vi "ScalePitchCtrl.vi"(6 "Scale Direction":T3=enum."Full scale -> Model scale", 8 "Scale Factor":dbl, 11 "PitchCtrl (In)":T1={"P-Gain"=0.0, "Blade pitch operating mode"=enum."From File", "Constant setpoint (deg)"=0.0, "I-Gain"=0.0, "Pitch from File (deg)"=0.0, "Homing vel (rpm)"=0.0, "Max vel (rpm)"=0.0, "Max vel change (rpm/min)"=0.0}) -> (3 "PitchCtrl (Out)":T1={"P-Gain"=0.0, "Blade pitch operating mode"=enum."From File", "Constant setpoint (deg)"=0.0, "I-Gain"=0.0, "Pitch from File (deg)"=0.0, "Homing vel (rpm)"=0.0, "Max vel (rpm)"=0.0, "Max vel change (rpm/min)"=0.0})   [LabVIEW 2018]
uses:
  Clusters/ScalingEnum.ctl
  Clusters/PitchCtrl.ctl
  Clusters/BladePitchMode.ctl
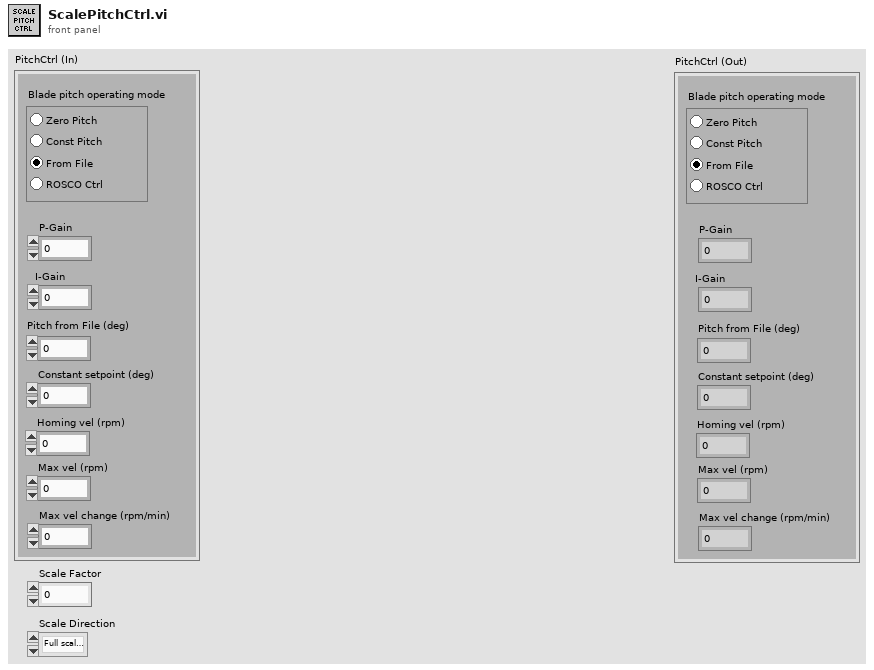
[diagram p1: front panel]
types:
  T1 = typedef "PitchCtrl.ctl" = cluster{"P-Gain":dbl, "Blade pitch operating mode":T2, "Constant setpoint (deg)":dbl, "I-Gain":dbl, "Pitch from File (deg)":dbl, "Homing vel (rpm)":dbl, "Max vel (rpm)":dbl, "Max vel change (rpm/min)":dbl}
  T2 = typedef "BladePitchMode.ctl" = enum32{"Zero pitch", "Const pitch", "From File", "ROSCO Ctrl"}
  T3 = typedef "ScalingEnum.ctl" = enum16{"Model scale -> Full scale", "Full scale -> Model scale"}
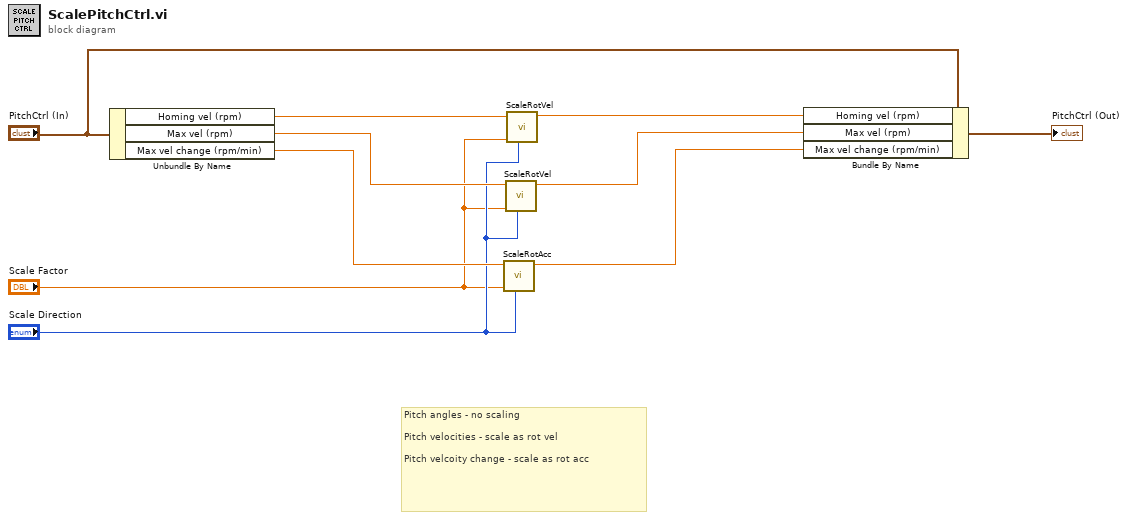
[diagram p0: block diagram]
diagram:
  # "Pitch angles - no scaling\n\nPitch velocities - scale as rot vel\n\nPitch velcoity change - scale as rot acc"
  n1 = Unbundle By Name("PitchCtrl (In)") -> ("Homing vel (rpm)"=w10:dbl, "Max vel (rpm)"=w7:dbl, "Max vel change (rpm/min)"=w5:dbl)
  n2 = call "ScaleRotAcc.vi"("Scale Dir"="Scale Direction", "Scale factor"="Scale Factor", "Rotational Acceleration (In)"=w5) -> ("Rotational Acceleration (Out)"=w2:dbl)  [unwired: 8 in]
  n3 = call "ScaleRotVel.vi"("Scale Dir"="Scale Direction", "Scale factor"="Scale Factor", "Rotational Velocity (In)"=w7) -> ("Rotational Velocity (Out)"=w6:dbl)  [unwired: 8 in]
  n4 = call "ScaleRotVel.vi"("Scale Dir"="Scale Direction", "Scale factor"="Scale Factor", "Rotational Velocity (In)"=w10) -> ("Rotational Velocity (Out)"=w8:dbl)  [unwired: 8 in]
  n5 = Bundle By Name(cluster="PitchCtrl (In)", "Homing vel (rpm)"=w8, "Max vel (rpm)"=w6, "Max vel change (rpm/min)"=w2) -> (→"PitchCtrl (Out)":T1)
